vi "ArcAndTheta.vi"(6 "Limit of Orientation Change":dbl=1.0, 7 "Amount of Time (s)":dbl=1.0, 8 "Absolute Theta Final":dbl, 9 "Absolute Theta initial":dbl, 10 "Y":dbl[](array[numeric]), 11 "X":dbl[](array[numeric])) -> (1 "Theta(arc length)":dbl[](array[numeric]), 2 "Arc Length":dbl[](array[numeric]), 3 "TimeStamp":dbl[](array[numeric]), 4 "Verify Graph":cluster{"X":dbl, "Y":dbl}[](graph))   [LabVIEW 2016]
uses:
  <vilib>/Analysis/1siggen.llb/Ramp Pattern by Samples.vi
  <vilib>/gmath/NI_Gmath.lvlib
  <vilib>/Analysis/NI_AALBase.lvlib
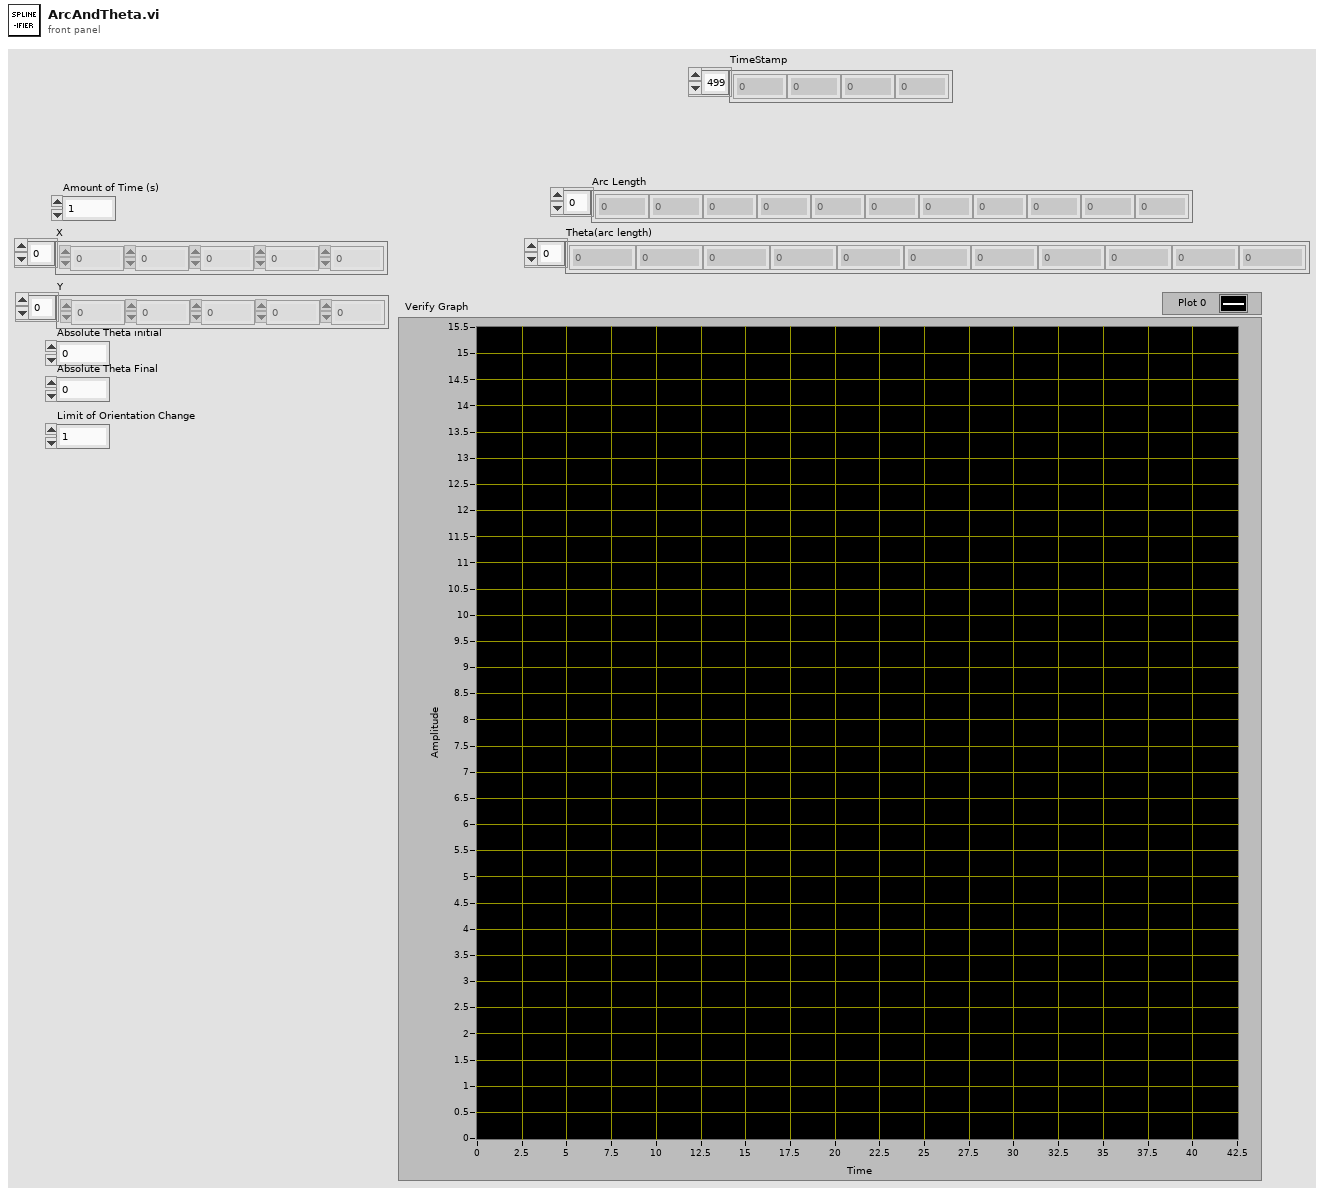
[diagram p1: front panel]
types:
  T1 = cluster{"boundary":enum16{"natural spline", "not-a-knot", "1st derivative", "2nd derivative"}, "derivative value":dbl}
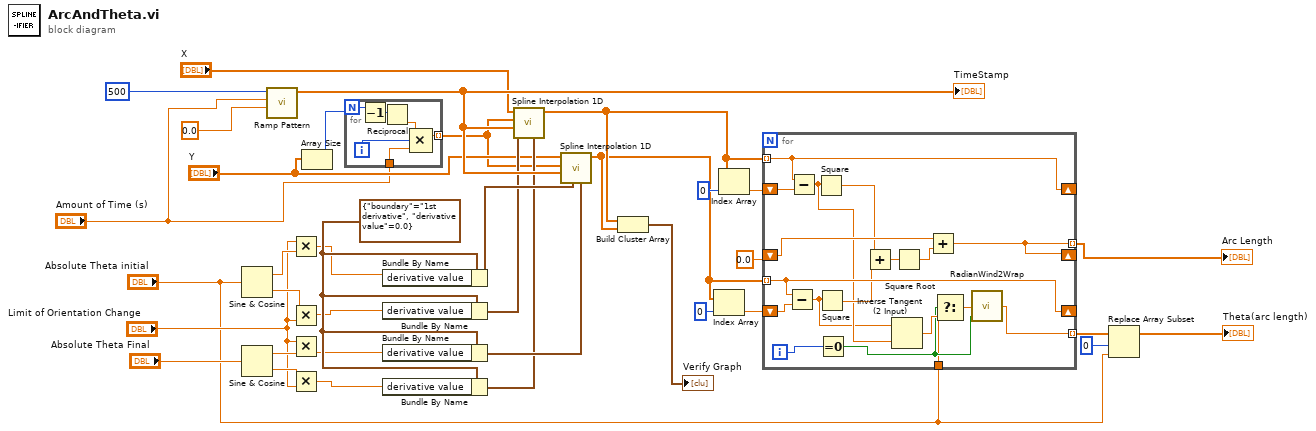
[diagram p0: block diagram]
diagram:
  w34 = T1 {"boundary"=enum."1st derivative", "derivative value"=0.0} ("initial boundary")
  n1 = Sine & Cosine(0:"Absolute Theta initial") -> (1:w18:dbl, 2:w20:dbl)
  n2 = Sine & Cosine(0:"Absolute Theta Final") -> (1:w16:dbl, 2:w14:dbl)
  n3 = call-poly <vilib>:"Ramp Pattern.vi"("start"=0.0, "end"="Amount of Time (s)", "samples"=500) -> ("Ramp Pattern"=w35:dbl[])  [unwired: 7 in, 1 out]
  "TimeStamp" <- w35
  n4 = Multiply(x="Limit of Orientation Change", y=w18) -> (x*y=w17:dbl)
  n5 = Multiply(x=w20, y="Limit of Orientation Change") -> (x*y=w19:dbl)
  n6 = Multiply(x="Limit of Orientation Change", y=w16) -> (x*y=w15:dbl)
  n7 = Multiply(x=w14, y="Limit of Orientation Change") -> (x*y=w13:dbl)
  n8 = Array Size(array="Y") -> (size(s)=w22:i32)
  n9 = for {
    N: w22 -> [w39]
    tunnel: [w40] -> w21 mode=indexing
    tunnel: "Amount of Time (s)" -> [w37]
    i -> [w41]
    n10 = Decrement(x=w39) -> (x-1=w38:i32)
    n11 = Reciprocal(x=w38) -> (1/x=w42:dbl)
    n12 = Compound Arithmetic op=MULTIPLY(w42, w41, w37) -> (w40:dbl)
  }
  n13 = Bundle By Name(cluster=w34, "derivative value"=w17) -> (w33:T1)
  n14 = Bundle By Name(cluster=w34, "derivative value"=w19) -> (w32:T1)
  n15 = Bundle By Name(cluster=w34, "derivative value"=w15) -> (w31:T1)
  n16 = Bundle By Name(cluster=w34, "derivative value"=w13) -> (w30:T1)
  n17 = call <vilib>:"Spline Interpolation 1D.vi"("final boundary"=w30, "initial boundary"=w32, "xi"=w35, "X"=w21, "Y"="X") -> ("yi"=w4:dbl[])  [unwired: 4 in, 2 out]
  n18 = call <vilib>:"Spline Interpolation 1D.vi"("final boundary"=w31, "initial boundary"=w33, "xi"=w35, "X"=w21, "Y"="Y") -> ("yi"=w3:dbl[])  [unwired: 4 in, 2 out]
  n19 = Build Cluster Array(w4, w3) -> (→"Verify Graph":cluster{"Numeric":dbl, "Numeric":dbl}[])
  n20 = Index Array(array=w3, index=0) -> (element=w28:dbl)
  n21 = Index Array(array=w4, index=0) -> (element=w27:dbl)
  n22 = for {
    tunnel: w3 -> [w59] mode=indexing
    tunnel: w4 -> [w57] mode=indexing
    shift-right: [w57] -> _
    shift-left: w27 -> [w58]
    shift-right: [w59] -> _
    shift-left: w28 -> [w60]
    tunnel: [w53] -> w6 mode=indexing
    tunnel: [w48] -> w10 mode=indexing
    shift-right: [w53] -> _
    shift-left: 0.0 -> [w52]
    tunnel: "Absolute Theta initial" -> [w43]
    i -> [w47]
    n23 = Subtract(x=w59, y=w60) -> (x-y=w49:dbl)
    n24 = Subtract(x=w57, y=w58) -> (x-y=w51:dbl)
    n25 = Square(x=w51) -> (x^2=w50:dbl)
    n26 = Square(x=w49) -> (x^2=w54:dbl)
    n27 = Equal To 0?(x=w47) -> (x = 0?=w44:bool)
    n28 = Add(x=w50, y=w54) -> (x+y=w56:dbl)
    n29 = Inverse Tangent (2 Input)(1:w51, 2:w49) -> (0:w46:dbl)
    n30 = Square Root(x=w56) -> (sqrt(x)=w55:dbl)
    n31 = Add(x=w52, y=w55) -> (x+y=w53:dbl)
    n32 = Select(t=w43, s=w44, f=w46) -> (s? t:f=w45:dbl)
    n33 = call "RadianWind2Wrap.vi"("Reset"=w44, "In"=w45) -> ("Out"=w48:dbl)  [unwired: 3 in]
  }
  "Arc Length" <- w6
  n34 = Replace Array Subset(array=w10, new element="Absolute Theta initial", index=0) -> (→"Theta(arc length)":dbl[])
